vi "TestSubVI.vi"(8 "Error In":errorcluster, 11 "Numeric":dbl) -> (0 "Error Out":errorcluster)   [LabVIEW 2018]
uses:
  TracerLibrary/Tracer/Tracer.lvclass
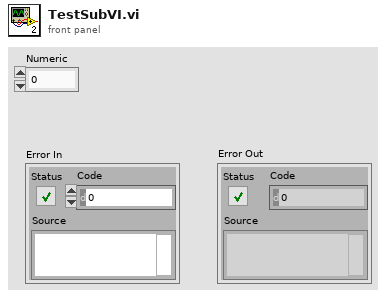
[diagram p1: front panel]
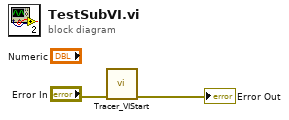
[diagram p0: block diagram]
diagram:
  n1 = call "Tracer_VIStart.vi"("Error In"="Error In") -> ("Error Out"=→"Error Out":errorcluster)  [unwired: 14 in]
